vi "Read Object.vi"(8 "error in (no error)":errorcluster, 11 "User in":refnum<class "User.lvclass">) -> (0 "error out":errorcluster, 2 "Object":string, 3 "User out":refnum<class "User.lvclass">)   [LabVIEW 2018, in "User.lvclass"]
doc: "Este VI faz a leitura do nome do objeto astronômico salvo na classe."
uses:
  User.lvclass
  User.lvclass/User.ctl
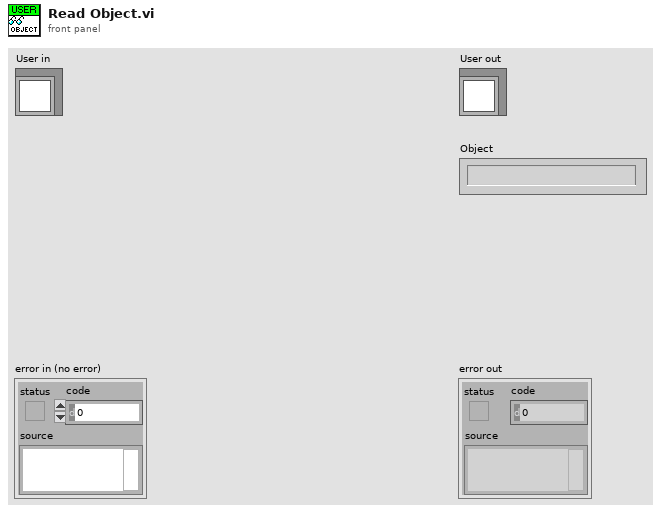
[diagram p1: front panel]
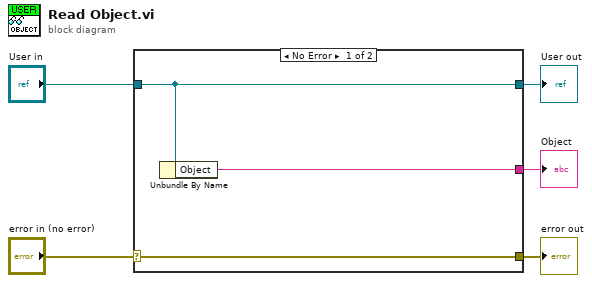
[diagram p0: block diagram]
diagram:
  n1 = case shown="No Error" "error in (no error)" {
    selector: "error in (no error)" -> [w8 w9]
    tunnel: [w8 w9] -> w4
    tunnel: [w7 w10] -> w2
    tunnel: "User in" -> [w7 w10]
    tunnel: [w6 _] -> w1
    frame No Error {
      n2 = Unbundle By Name(w7) -> ("Object"=w6:string)
    }
    frame Error {
    }
  }
  "error out" <- w4
  "User out" <- w2
  "Object" <- w1
